vi "verify result.vi"(0 "comparison":T1 caption="Enum", 1 "Skip test?":bool, 5 "measured data":dbl format="%#_13g", 7 "UL":dbl format="%#_13g", 9 "LL":dbl format="%#_13g", 11 "error in (no error)":errorcluster) -> (4 "measured value":string, 6 "result":string, 10 "result?":bool, 15 "error out":errorcluster)   [LabVIEW 2022 SP3]
uses:
  controls/comparison selection.ctl
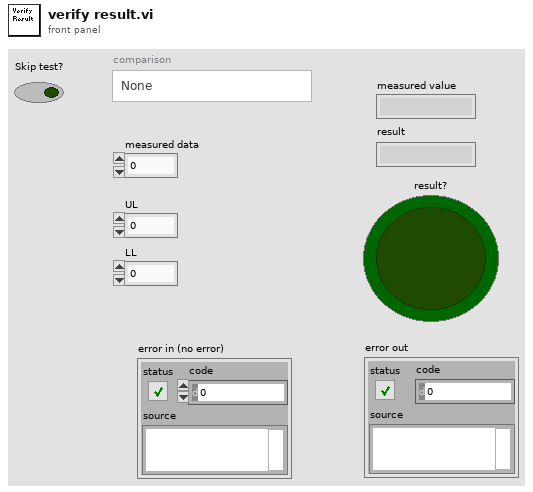
[diagram p1: front panel]
types:
  T1 = typedef "comparison selection.ctl" = enum16{"None", "in-range?", "less than?", "greater than?", "equal to?", "not equal to?", "less or equal to?", "greater or equal to?"}
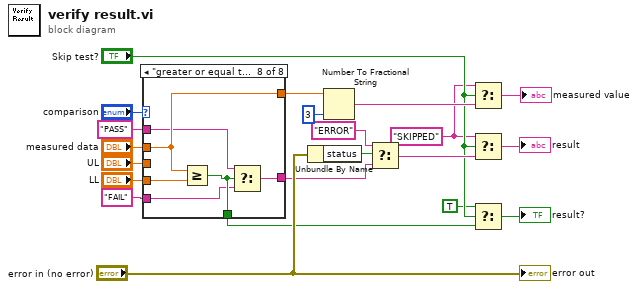
[diagram p0: block diagram]
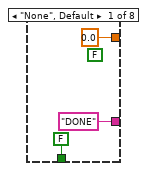
[diagram p2: hidden frame]
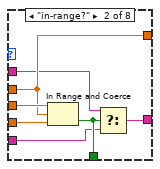
[diagram p3: hidden frame]
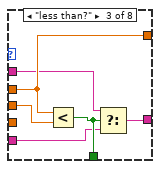
[diagram p4: hidden frame]
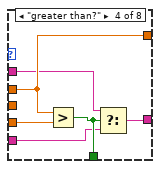
[diagram p5: hidden frame]
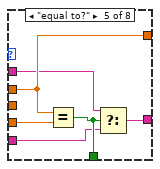
[diagram p6: hidden frame]
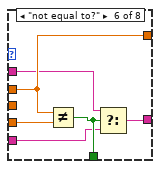
[diagram p7: hidden frame]
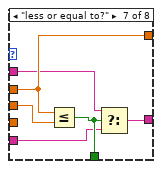
[diagram p8: hidden frame]
diagram:
  w3 = "SKIPPED" ("f")
  n1 = case shown="\"greater or equal to?\"" "comparison" {
    tunnel: ["DONE" ("f") w29 w37 w42 w48 w54 w61 w66] -> w14
    tunnel: "UL" -> [_ w31 w32 _ _ _ w56 _]
    tunnel: "LL" -> [_ w30 _ w43 w49 w55 _ w67]
    tunnel: "measured data" -> [_ w27 w35 w40 w46 w52 w59 w64]
    tunnel: [FALSE w28 w36 w41 w47 w53 w60 w65] -> w8
    tunnel: [0.0 ("Measured Data") w27 w35 w40 w46 w52 w59 w64] -> w12
    tunnel: "PASS" ("t") -> [_ w26 w34 w38 w45 w51 w58 w63]
    tunnel: "FAIL" ("f") -> [_ w25 w33 w39 w44 w50 w57 w62]
    frame "None", Default {
      (unwired) FALSE
    }
    frame "in-range?" {
      n2 = In Range and Coerce(upper limit=w31, x=w27, lower limit=w30) -> (In Range?=w28:bool)  [unwired: 1 out]
      n3 = Select(t=w26, s=w28, f=w25) -> (s? t:f=w29:string)
    }
    frame "less than?" {
      n4 = Less?(x=w35, y=w32) -> (x < y?=w36:bool)
      n5 = Select(t=w34, s=w36, f=w33) -> (s? t:f=w37:string)
    }
    frame "greater than?" {
      n6 = Greater?(x=w40, y=w43) -> (0:w41:bool)
      n7 = Select(t=w38, s=w41, f=w39) -> (s? t:f=w42:string)
    }
    frame "equal to?" {
      n8 = Equal?(x=w46, y=w49) -> (x = y?=w47:bool)
      n9 = Select(t=w45, s=w47, f=w44) -> (s? t:f=w48:string)
    }
    frame "not equal to?" {
      n10 = Not Equal?(x=w52, y=w55) -> (x != y?=w53:bool)
      n11 = Select(t=w51, s=w53, f=w50) -> (s? t:f=w54:string)
    }
    frame "less or equal to?" {
      n12 = Less Or Equal?(x=w59, y=w56) -> (x <= y?=w60:bool)
      n13 = Select(t=w58, s=w60, f=w57) -> (s? t:f=w61:string)
    }
    frame "greater or equal to?" {
      n14 = Greater Or Equal?(x=w64, y=w67) -> (x >= y?=w65:bool)
      n15 = Select(t=w63, s=w65, f=w62) -> (s? t:f=w66:string)
    }
  }
  n16 = Unbundle By Name("error in (no error)") -> ("status"=w16:bool)
  n17 = Number To Fractional String(number=w12, precision (6)=i16 3) -> (F-format string=w10:string)  [unwired: 2 in]
  n18 = Select(t="ERROR" ("message"), s=w16, f=w14) -> (s? t:f=w13:string)
  n19 = Select(t=w3, s="Skip test?", f=w10) -> (s? t:f=→"measured value":string)
  n20 = Select(t=w3, s="Skip test?", f=w13) -> (s? t:f=→"result":string)
  n21 = Select(t=TRUE, s="Skip test?", f=w8) -> (s? t:f=→"result?":bool)
  "error out" <- "error in (no error)"
